vi "Get 1 Pin Object.vi"(8 "error in":errorcluster, 10 "pin or relay name":string, 11 "session reservation in":refnum<class "Session Reservation.lvclass">) -> (0 "error out":errorcluster, 2 "instrument object":refnum<class "DMM_Base.lvclass">, 3 "session reservation out":refnum<class "Session Reservation.lvclass">)   [LabVIEW 2021, in "DMM_Base.lvclass"]
doc: "Gets a single pin_name and gives a LabVIEW object for it. The LabVIEW object is then typecasted to the DMM_Base class object and is updated with the session reservation, pin_name and the channel information."
uses:
  DMM_Base.lvclass
  <vilib>/Plug-In SDKs/Clients/Session Management V1/Session Reservation/Session Reservation.lvclass
  Reusables/Get Pin Information.lvlib
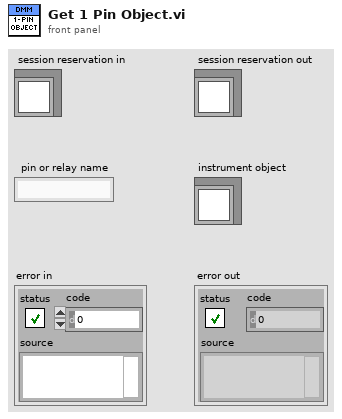
[diagram p1: front panel]
types:
  T1 = typedef "ni.measurementlink.sessionmanagement.v1.api.lvlib/ni_measurementlink_sessionmanagement_v1_ChannelMapping.ctl" = cluster{"pin_or_relay_name":string, "site":i32, "channel":string, "multiplexer_resource_name":string, "multiplexer_route":string}
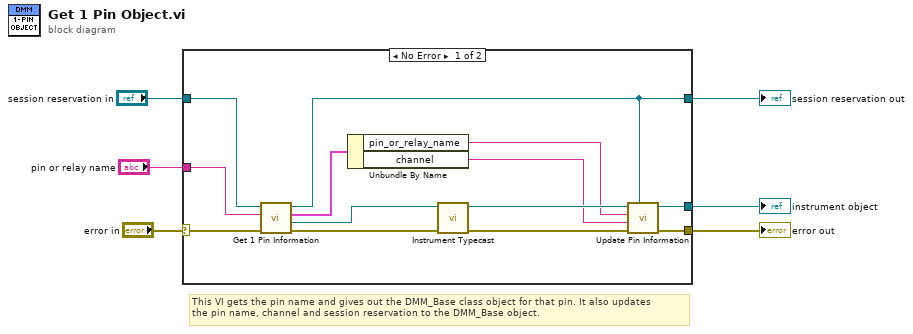
[diagram p0: block diagram]
diagram:
  # "This VI gets the pin name and gives out the DMM_Base class object for that pin. It also updates\nthe pin name, channel and session reservation to the DMM_Base object."
  n1 = case shown="No Error" "error in" {
    selector: "error in" -> [w17 w21]
    tunnel: "session reservation in" -> [w19 w20]
    tunnel: "pin or relay name" -> [w18 _]
    tunnel: [w10 w21] -> w3
    tunnel: [w9 _] -> w2
    tunnel: [w8 w20] -> w1
    frame No Error {
      n2 = call "Get 1 Pin Information.vi"("error in"=w17, "pin or relay name"=w18, "session reservation in"=w19) -> ("error out"=w14:errorcluster, "pin instrument"=w7:refnum<class>, "channel_mapping"=w16:T1, "session reservation out"=w8:refnum<class "Session Reservation.lvclass">)  [unwired: 5 in]
      n3 = Unbundle By Name(w16) -> ("pin_or_relay_name"=w11:string, "channel"=w12:string)
      n4 = call "Instrument Typecast.vi"("error in (no error)"=w14, "pin instrument"=w7) -> ("error out"=w15:errorcluster, "instrument object"=w13:refnum<class "DMM_Base.lvclass">)  [unwired: 8 in]
      n5 = call "Update Pin Information.vi"("Session Reservation"=w8, "error in"=w15, "channel"=w12, "pin_name"=w11, "instrument object in"=w13) -> ("error out"=w10:errorcluster, "instrument object out"=w9:refnum<class "DMM_Base.lvclass">)  [unwired: 5 in]
    }
    frame Error {
    }
  }
  "session reservation out" <- w1
  "error out" <- w3
  "instrument object" <- w2
